vi "Get MeasData Q and Insert Logging Data.vi"(7 "bypass":bool, 8 "error in":errorcluster) -> (0 "error out":errorcluster, 2 "MeasData out":T1, 5 "# elements in queue":i32)   [LabVIEW 2017]
doc: "Developed by Kevin Thompson\nThompson Engineering, LLC\nkevin@thompsonengineering.net"
uses:
  TD MeasData--cluster.ctl
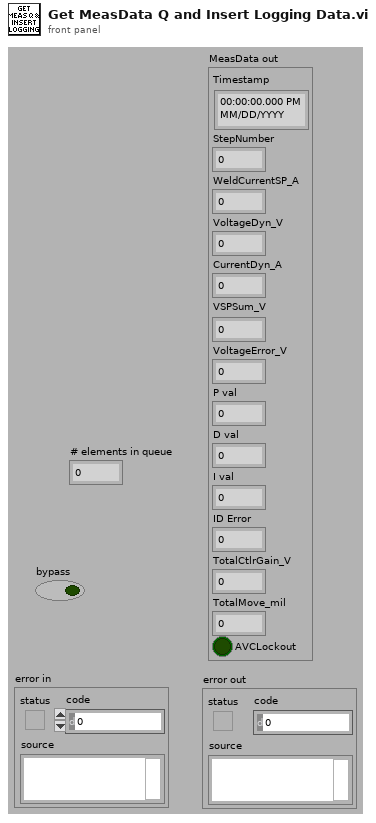
[diagram p1: front panel]
types:
  T1 = typedef "TD MeasData--cluster.ctl" = cluster{"Timestamp":timestamp, "StepNumber":i32, "WeldCurrentSP_A":dbl, "VoltageDyn_V":dbl, "CurrentDyn_A":dbl, "VSPSum_V":dbl, "VoltageError_V":dbl, "P val":dbl, "D val":dbl, "I val":dbl, "ID Error":dbl, "TotalCtlrGain_V":dbl, "TotalMove_mil":dbl, "AVCLockout":bool}
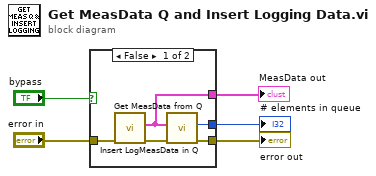
[diagram p0: block diagram]
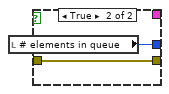
[diagram p2: hidden frame]
diagram:
  n1 = case shown="False" "bypass" {
    tunnel: [w10 w12] -> w5
    tunnel: "error in" -> [w8 w12]
    tunnel: [w7 _] -> w2
    tunnel: [w6 w11] -> w1
    frame False {
      n2 = call "Get MeasData from Q.vi"("error in (no error)"=w8) -> ("error out"=w9:errorcluster, "MeasData out"=w7:T1)  [unwired: 8 in, 1 out]
      n3 = call "Insert LogMeasData in Q.vi"("error in (no error)"=w9, "MeasData"=w7) -> ("error out"=w10:errorcluster, "# elements in queue"=w6:i32)  [unwired: 7 in, 1 out]
    }
    frame True {
      n4 = local read "# elements in queue"() -> (w11:i32)
    }
  }
  "error out" <- w5
  "MeasData out" <- w2
  "# elements in queue" <- w1
